vi "Write Initial Data Serial Number.vi"(8 "error in (no error)":errorcluster, 10 "Initial Data Serial Number":u32, 11 "Micron sm Digitizer in":refnum<class "Micron sm Digitizer.lvclass">) -> (0 "error out":errorcluster, 3 "Micron sm Digitizer out":refnum<class "Micron sm Digitizer.lvclass">)   [LabVIEW 2024, in "Micron sm Digitizer.lvclass"]
uses:
  Micron sm Digitizer.lvclass
  Micron sm Digitizer.lvclass/Micron sm Digitizer.ctl
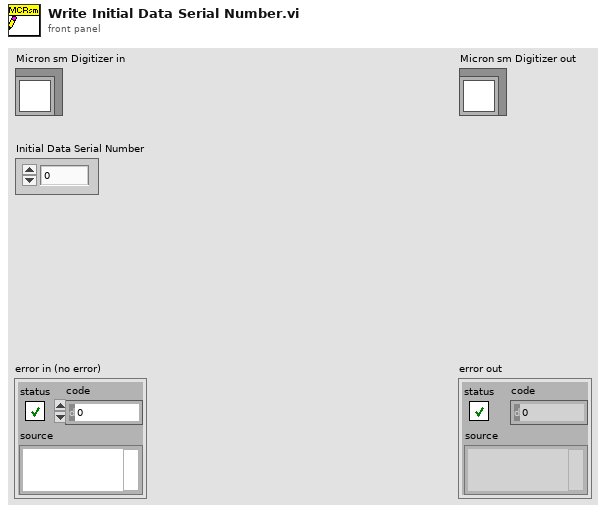
[diagram p1: front panel]
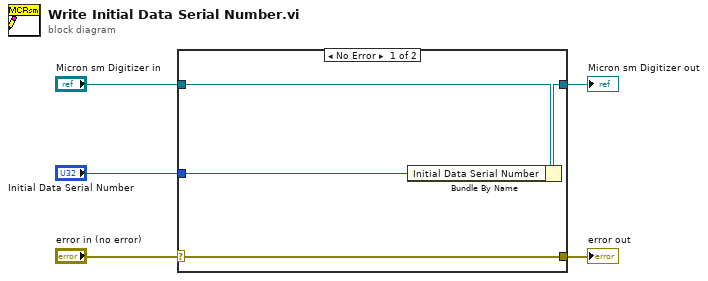
[diagram p0: block diagram]
diagram:
  n1 = case shown="No Error" "error in (no error)" {
    selector: "error in (no error)" -> [w9 w10]
    tunnel: [w9 w10] -> w4
    tunnel: [w7 w11] -> w2
    tunnel: "Micron sm Digitizer in" -> [w8 w11]
    tunnel: "Initial Data Serial Number" -> [w6 _]
    frame No Error {
      n2 = Bundle By Name(cluster=w8, "Initial Data Serial Number"=w6) -> (w7:refnum<class "Micron sm Digitizer.lvclass">)
    }
    frame Error {
    }
  }
  "error out" <- w4
  "Micron sm Digitizer out" <- w2
